vi "Transport.vi"(5 "LogSuspend":bool, 8 "error in":errorcluster, 10 "Request":string="19 02 08", 11 "UdsHandleIn":T1={"LogPath"=path "", "LogEnabled"=FALSE, "isOpen"=FALSE, "LogContent"="", "Adapter"="CAN0", "MCanHandle"={"MCanAdapter"=refnum}, "TransmittId"=0, "ReceiveId"=0}) -> (0 "error out":errorcluster, 2 "Response":string, 3 "UdsHandleOut":T1={"LogPath"=path "", "LogEnabled"=FALSE, "isOpen"=FALSE, "LogContent"="", "Adapter"="CAN0", "MCanHandle"={"MCanAdapter"=refnum}, "TransmittId"=0, "ReceiveId"=0})   [LabVIEW 2011, in "Konvolucio MUDS150628.lvlib"]
uses:
  <instrlib>/Konvolucio MUDS150628/Konvolucio MUDS150628.lvlib
  <instrlib>/Konvolucio MUDS150628/Types/UdsHandleType.ctl
  <instrlib>/Konvolucio MCAN120803/Types/MCanHandleType.ctl
  C:/Program Files/National Instruments/LabVIEW 2011/instr.lib/Konvolucio MCAN120803/Private/Konvolucio.MCAN120803.dll
  Konvolucio MCAN120803/Private/Konvolucio.MCAN120803.dll
  <instrlib>/Konvolucio MCAN120803/Konvolucio MCAN120803.lvlib
panel:
  out "NaN/Path/Refnum?":bool
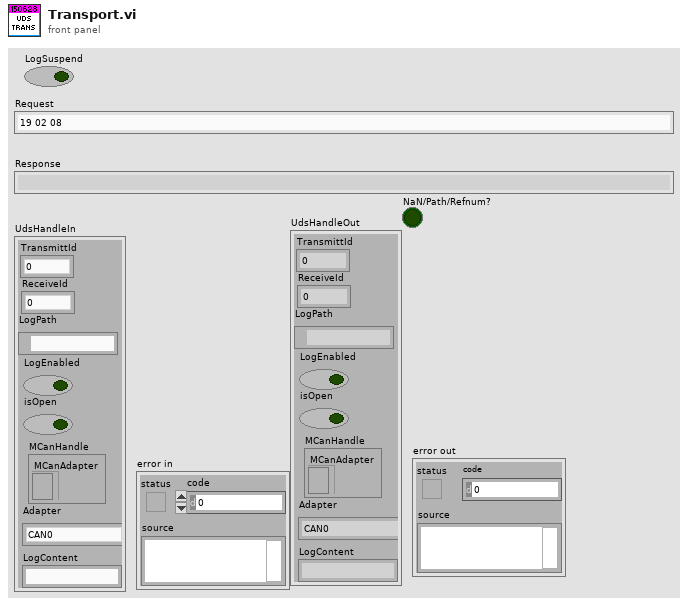
[diagram p1: front panel]
types:
  T1 = typedef "Konvolucio MUDS150628.lvlib/UdsHandleType.ctl" = cluster{"LogPath":path, "LogEnabled":bool, "isOpen":bool, "LogContent":string, "Adapter":string, "MCanHandle":T2, "TransmittId":u32, "ReceiveId":u32}
  T2 = typedef "Konvolucio MCAN120803.lvlib/MCanHandleType.ctl" = cluster{"MCanAdapter":refnum<k24>}
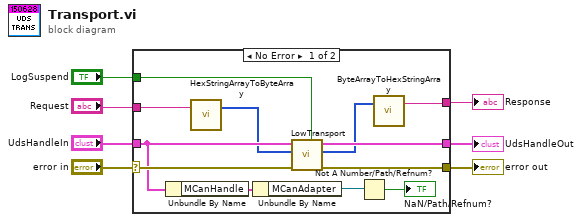
[diagram p0: block diagram]
diagram:
  n1 = case shown="No Error" "error in" {
    selector: "error in" -> [w16 w21]
    tunnel: "Request" -> [w11 w22]
    tunnel: [w8 w22] -> w6
    tunnel: "UdsHandleIn" -> [w15 w20]
    tunnel: [w19 w20] -> w4
    tunnel: [w18 w21] -> w3
    tunnel: "LogSuspend" -> [w17 _]
    frame No Error {
      n2 = Unbundle By Name(w15) -> ("MCanHandle"=w14:T2)
      n3 = call <instrlib>:"HexStringArrayToByteArray.vi"("HexStirngArray"=w11) -> ("ByteArrayOut"=w10:u8[])  [unwired: 2 in]
      n4 = Unbundle By Name(w14) -> ("MCanAdapter"=w13:refnum<k24>)
      n5 = call <instrlib>:"LowTransport.vi"("LogSuspend"=w17, "error in"=w16, "Request"=w10, "HandleIn"=w15) -> ("error out"=w18:errorcluster, "Response"=w9:u8[], "HandleOut"=w19:T1)  [unwired: 5 in]
      n6 = Not A Number/Path/Refnum?(number/path/refnum=w13) -> (NaN/Path/Refnum?=→"NaN/Path/Refnum?":bool)
      n7 = call <instrlib>:"ByteArrayToHexStringArray.vi"("ByteArrayIn"=w9) -> ("HexStringArrayOut"=w8:string)  [unwired: 2 in]
    }
    frame Error {
    }
  }
  "Response" <- w6
  "UdsHandleOut" <- w4
  "error out" <- w3
